vi "Shuffle Array 2D Template.vi"(0 "Array In":variant[][](array[variant]), 1 "Rank":enum16{"Rows", "Columns", "Both"}(ring)) -> (2 "Shuffled Array":variant[][](array[variant]))   [LabVIEW 2018]
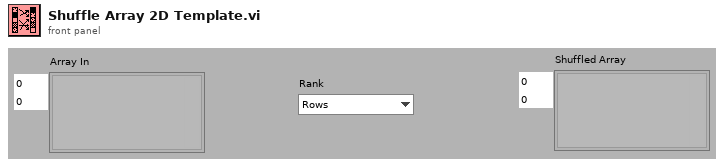
[diagram p1: front panel]
types:
  T1 = cluster{"number: 0 to 1":dbl, "Array In":variant[]}
  T2 = cluster{"number: 0 to 1":dbl, "Array In":variant[]}[]
  T3 = cluster{"number: 0 to 1":dbl, "Variant":variant}[]
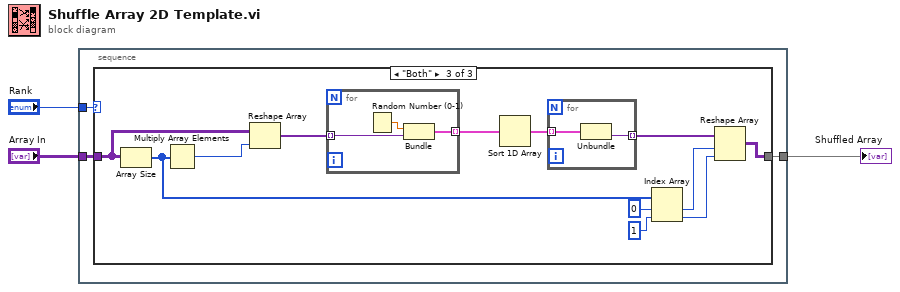
[diagram p0: block diagram]
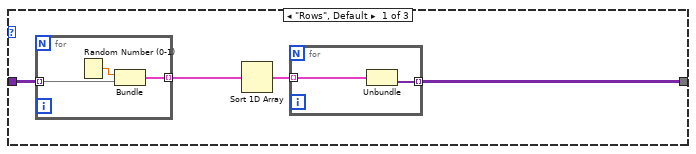
[diagram p2: hidden frame]
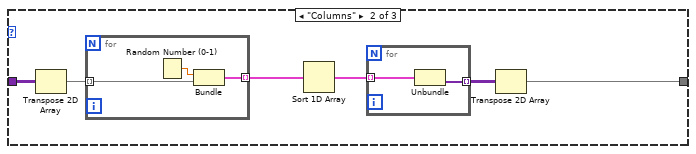
[diagram p3: hidden frame]
diagram:
  n1 = stacked-sequence {
    tunnel: "Array In" -> [w6]
    tunnel: [w5] -> w2
    tunnel: "Rank" -> [w4]
    frame #0 {
      n2 = case shown="\"Both\"" w4 {
        tunnel: w6 -> [w10 w21 w35]
        tunnel: [w7 w16 w32] -> w5
        frame "Rows", Default {
          n3 = for {
            tunnel: w10 -> [w14] mode=indexing
            tunnel: [w13] -> w9 mode=indexing
            n4 = Random Number (0-1)() -> (number: 0 to 1=w15:dbl)
            n5 = Bundle("number: 0 to 1"=w15, "Array In"=w14) -> (w13:T1)  [unwired: 1 out]
          }
          n6 = Sort 1D Array(array=w9) -> (sorted array=w8:T2)
          n7 = for {
            tunnel: w8 -> [w12] mode=indexing
            tunnel: [w11] -> w7 mode=indexing
            n8 = Unbundle(w12) -> ("Array In"=w11:variant[])  [unwired: 1 out]
          }
        }
        frame "Columns" {
          n9 = Transpose 2D Array(2D array=w21) -> (transposed array=w17:variant[][])
          n10 = for {
            tunnel: w17 -> [w25] mode=indexing
            tunnel: [w24] -> w20 mode=indexing
            n11 = Random Number (0-1)() -> (number: 0 to 1=w26:dbl)
            n12 = Bundle("number: 0 to 1"=w26, w25) -> (w24:cluster{"number: 0 to 1":dbl, variant[]})  [unwired: 1 out]
          }
          n13 = Sort 1D Array(array=w20) -> (sorted array=w19:cluster{"number: 0 to 1":dbl, variant[]}[])
          n14 = for {
            tunnel: w19 -> [w23] mode=indexing
            tunnel: [w22] -> w18 mode=indexing
            n15 = Unbundle(w23) -> (w22:variant[])  [unwired: 1 out]
          }
          n16 = Transpose 2D Array(2D array=w18) -> (transposed array=w16:variant[][])
        }
        frame "Both" {
          n17 = Array Size(array=w35) -> (size(s)=w31:i32[])
          n18 = Multiply Array Elements(1:w31) -> (0:w36:i32)
          n19 = Reshape Array(w35, w36) -> (w34:variant[])
          n20 = for {
            tunnel: w34 -> [w42] mode=indexing
            tunnel: [w41] -> w38 mode=indexing
            n21 = Random Number (0-1)() -> (number: 0 to 1=w43:dbl)
            n22 = Bundle("number: 0 to 1"=w43, "Variant"=w42) -> (w41:cluster{"number: 0 to 1":dbl, "Variant":variant})  [unwired: 1 out]
          }
          n23 = Sort 1D Array(array=w38) -> (sorted array=w37:T3)
          n24 = for {
            tunnel: w37 -> [w40] mode=indexing
            tunnel: [w39] -> w33 mode=indexing
            n25 = Unbundle(w40) -> ("Variant"=w39:variant)  [unwired: 1 out]
          }
          n26 = Index Array(array=w31, index #1=0 ("index"), index #2=1 ("index")) -> (element #1=w28:i32, element #2=w27:i32)
          n27 = Reshape Array(w33, w28, w27) -> (w32:variant[][])
        }
      }
    }
  }
  "Shuffled Array" <- w2
